vi "checkStiffnessOutOfRange.vi"(8 "error in (no error)":errorcluster, 11 "StiffnessMonitor in":refnum<class "StiffnessMonitor.lvclass">) -> (0 "error out":errorcluster, 2 "stiffnessOutOfRangeIsTrue":bool, 3 "StiffnessMonitor out":refnum<class "StiffnessMonitor.lvclass">)   [LabVIEW 2013, in "StiffnessMonitor.lvclass"]
uses:
  StiffnessMonitor.lvclass
  StiffnessMonitor.lvclass/StiffnessMonitor.ctl
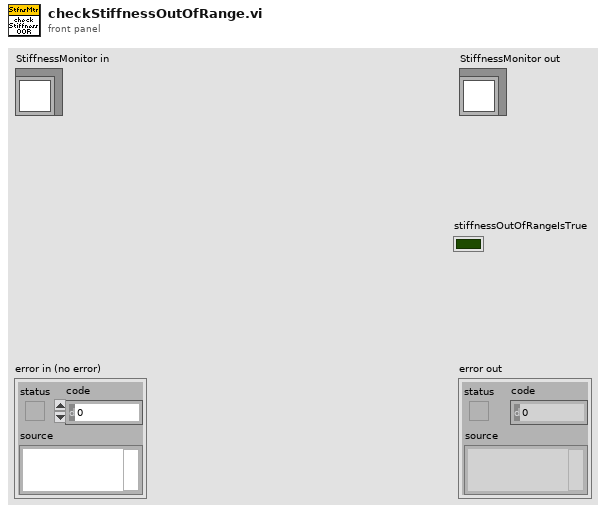
[diagram p1: front panel]
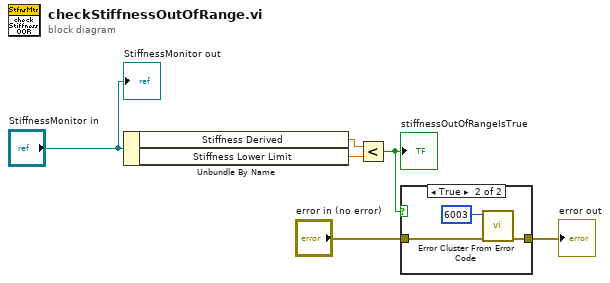
[diagram p0: block diagram]
diagram:
  n1 = Unbundle By Name("StiffnessMonitor in") -> ("Stiffness Derived"=w5:dbl[unit], "Stiffness Lower Limit"=w4:dbl[unit])
  n2 = Less?(x=w5, y=w4) -> (x < y?=w1:bool)
  "stiffnessOutOfRangeIsTrue" <- w1
  n3 = case shown="True" w1 {
    tunnel: "error in (no error)" -> [w7 w10]
    tunnel: [w7 w9] -> w2
    frame False {
    }
    frame True {
      n4 = call <vilib>:"Error Cluster From Error Code.vi"("error in (no error)"=w10, "error code (0)"=6003) -> ("error out"=w9:errorcluster)  [unwired: 7 in]
    }
  }
  "error out" <- w2
  "StiffnessMonitor out" <- "StiffnessMonitor in"
